vi "Read Container By Bitfield.vi"(8 "error in (no error)":errorcluster, 10 "Bitfield":u16, 11 "Storage Line in":refnum<class "Storage Line.lvclass">) -> (0 "error out":errorcluster, 1 "Containers":T1[](array[typedef]), 2 "Samples":refnum<class "Sample.lvclass">[](array[class]), 3 "Storage Line out":refnum<class "Storage Line.lvclass">, 5 "Indice":i32[](array[numeric]))   [LabVIEW 2015, in "cRIO-Carbondioxide.lvlib" / "CO2-Actor.lvlib" / "Storage Line.lvclass"]
uses:
  Storage Line.lvclass
  subs/Sample/Sample.lvclass
  Controls/Sample Container.ctl
  Storage Line.lvclass/Storage Line.ctl
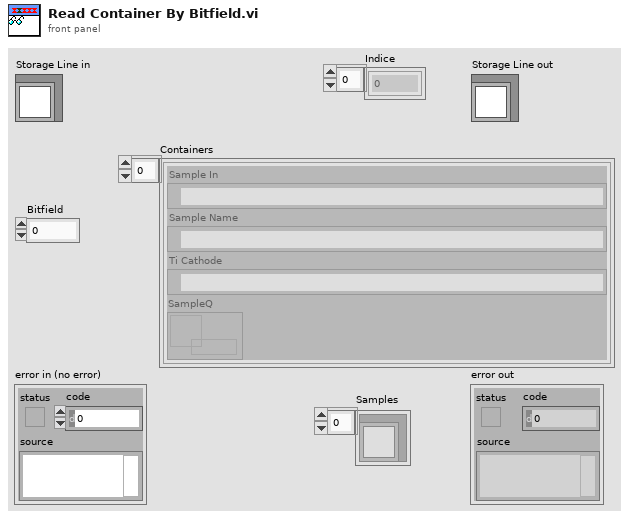
[diagram p1: front panel]
types:
  T1 = typedef "Sample Container.ctl" = cluster{"Sample In":refnum<k21>, "Sample Name":refnum<k21>, "Ti Cathode":refnum<k21>, "SampleQ":refnum<queue>}
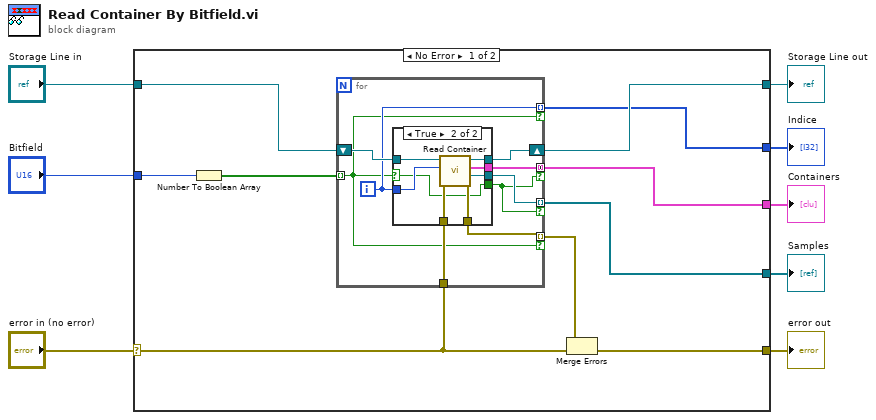
[diagram p0: block diagram]
diagram:
  n1 = case shown="No Error" "error in (no error)" {
    selector: "error in (no error)" -> [w16 w38]
    tunnel: [w13 w38] -> w7
    tunnel: [w14 w39] -> w5
    tunnel: "Storage Line in" -> [w15 w39]
    tunnel: "Bitfield" -> [w18 _]
    tunnel: [w10 _] -> w3
    tunnel: [w12 _] -> w2
    tunnel: [w9 _] -> w1
    frame No Error {
      n2 = Number To Boolean Array(number=w18) -> (Boolean array=w17:bool[])
      n3 = for {
        shift-right: [w26] -> w14
        shift-left: w15 -> [w27]
        tunnel: w17 -> [w19] mode=indexing
        tunnel: w16 -> [w25]
        tunnel: [w24] -> w11 mode=indexing if=w19
        tunnel: [w23] -> w10 mode=indexing if=w21
        tunnel: [w22] -> w12 mode=concatenating if=w21
        tunnel: [w20] -> w9 mode=indexing if=w19
        i -> [w20]
        n4 = case shown="True" w19 {
          selector: w19 -> [_ w31]
          tunnel: w27 -> [w29 w37]
          tunnel: [w29 w36] -> w26
          tunnel: w20 -> [_ w35]
          tunnel: w25 -> [w28 w34]
          tunnel: [w28 w33] -> w24
          tunnel: [_ w32] -> w23
          tunnel: [_ w31] -> w21
          tunnel: [_ w30] -> w22
          frame False {
          }
          frame True {
            n5 = call "Read Container.vi"("error in (no error)"=w34, "index"=w35, "Storage Line in"=w37) -> ("error out"=w33:errorcluster, "Sample out"=w32:refnum<class "Sample.lvclass">, "Containers"=w30:T1[], "Storage Line out"=w36:refnum<class "Storage Line.lvclass">)  [unwired: 5 in]
          }
        }
      }
      n6 = Merge Errors(w11, w16) -> (w13:errorcluster)
    }
    frame Error {
    }
  }
  "error out" <- w7
  "Storage Line out" <- w5
  "Samples" <- w3
  "Containers" <- w2
  "Indice" <- w1
